vi "Write O3 Flag.vi"(8 "error in":errorcluster, 10 "O3 Flag":bool, 11 "CRDS Data in":refnum<class "CRDS Data.lvclass">=refnum) -> (0 "error out":errorcluster, 3 "CRDS Data out":refnum<class "CRDS Data.lvclass">)   [LabVIEW 2012, in "CRDS Data.lvclass"]
uses:
  CRDS Data.lvclass
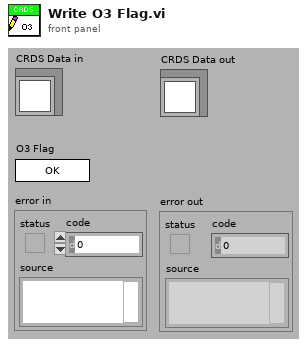
[diagram p1: front panel]
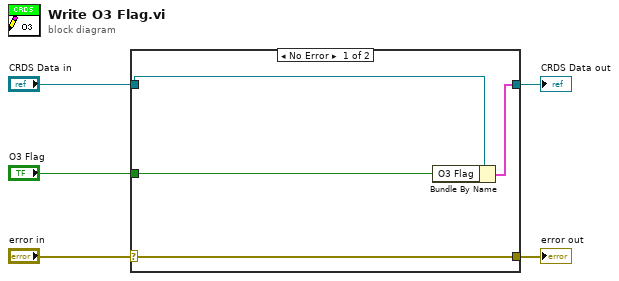
[diagram p0: block diagram]
diagram:
  n1 = case shown="No Error" "error in" {
    selector: "error in" -> [w9 w10]
    tunnel: [w9 w10] -> w4
    tunnel: [w7 w11] -> w2
    tunnel: "CRDS Data in" -> [w8 w11]
    tunnel: "O3 Flag" -> [w6 _]
    frame No Error {
      n2 = Bundle By Name(cluster=w8, "O3 Flag"=w6) -> (w7:cluster{})
    }
    frame Error {
    }
  }
  "error out" <- w4
  "CRDS Data out" <- w2
